vi "Close.vi"(11 "Custom Device in":refnum<class "NIDMM Engine.lvclass">) -> (0 "error out":errorcluster, 3 "Custom Device out":refnum<class "NIDMM Engine.lvclass">)   [LabVIEW 2026, in "NIDMM Engine.lvlib" / "NIDMM Engine.lvclass"]
uses:
  NIDMM Engine.lvclass
  NIDMM Engine.lvclass/NIDMM Engine.ctl
  <userlib>/NIVS Inline Async API (Express)/_VS Inline Async API (Express)/VS Inline Async API (Express)/VS Inline Async API (Express).lvclass
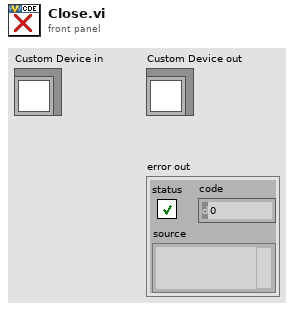
[diagram p1: front panel]
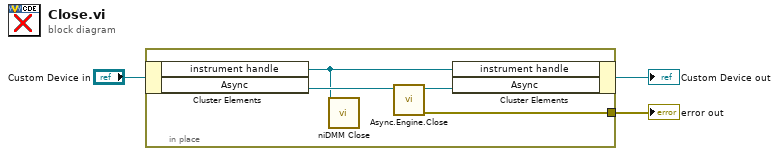
[diagram p0: block diagram]
diagram:
  n1 = in-place {
    in-place-border: [w7] -> w1
    n2 = in-place-cluster #1("Custom Device in") -> ("instrument handle"=w4:refnum<k15>, "Async"=w6:refnum<class "VS Inline Async API (Express).lvclass">)
    n3 = call <instrlib>:"niDMM Close.vi"("instrument handle"=w4) -> ()  [unwired: 10 in, 1 out]
    n4 = call <userlib>:"Async.Engine.Close.vi"("Async in"=w6) -> ("error out"=w7:errorcluster, "Async out"=w5:refnum<class "VS Inline Async API (Express).lvclass">)  [unwired: 9 in]
    n5 = in-place-cluster #1("instrument handle"=w4, "Async"=w5) -> (→"Custom Device out":refnum<class "NIDMM Engine.lvclass">)
  }
  "error out" <- w1
